vi "Untitled 3.vi"   [LabVIEW 2015]
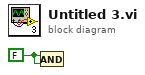
[diagram p0: block diagram]
diagram:
  w1 = FALSE ("x")
  n1 = And(x=w1, y=w1) -> ()  [unwired: 1 out]
